vi "(SubVI) Notch Filter for X Axis.vi"(0 "Sampling rate (Hz)":i32, 2 "Notch Filter On?":bool, 3 "data":dbl[](array[numeric])) -> (6 "Filtered Data":dbl[](array[numeric]))   [LabVIEW 2014]
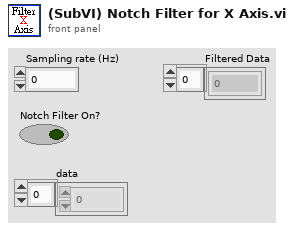
[diagram p1: front panel]
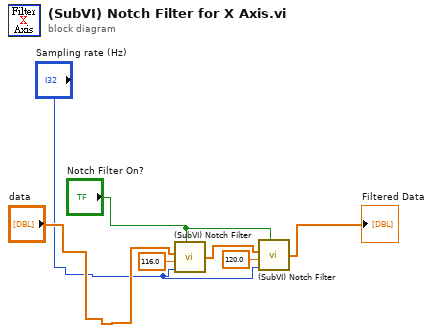
[diagram p0: block diagram]
diagram:
  n1 = call "(SubVI) Notch Filter.vi"("Notch Filter On?"="Notch Filter On?", "Data"="data", "Notch freq. (Hz)"=116.0, "Sampling rate (Hz)"="Sampling rate (Hz)") -> ("Filtered Data"=w3:dbl[])  [unwired: 4 in]
  n2 = call "(SubVI) Notch Filter.vi"("Notch Filter On?"="Notch Filter On?", "Data"=w3, "Notch freq. (Hz)"=120.0, "Sampling rate (Hz)"="Sampling rate (Hz)") -> ("Filtered Data"=→"Filtered Data":dbl[])  [unwired: 4 in]
